vi "PH_Beckhoff_StepMot.constructor.vi"(0 "name":string, 2 "data in":string, 5 "error in(no error)":errorcluster) -> (14 "i ref out":refnum<vi>, 16 "data out":string, 19 "error out":errorcluster)   [LabVIEW 2014, in "PH_Beckhoff_StepMot.lvlib"]
doc: "This is the constructor of a class.\n\nLicense Agreement for this software:\n\nCopyright (C)\nGesellschaft für Schwerionenforschung, GSI\nPlanckstr. 1\n64291 Darmstadt\nGermany\n\nContact: D.Beck@gsi.de \n\nThis program is free software; you can redistribute it and/or modify it under the terms of the \nGNU General Public License as published by the Free Software Foundation; either version 2 of \nthe license, or (at your option) any later version.\n\nThis program is distributed in the hope that it will be useful, but WITHOUT ANY WARRANTY; \nwithout even the implied warranty of MERCHANTABILITY or FITNESS FOR A PARTICULAR PURPOSE. See the GNU General License for more details (http://www.gnu.org).\n\nGesellschaft für Schwerionenforschung, GSI\nPlanckstr. 1, 64291 Darmstadt, Germany\nFor all questions and ideas contact: M.Richter@gsi.de, H.Brand@gsi.de or D.Beck@gsi.de.\nLast update: 16-JUN-2004"
uses:
  PH_Beckhoff_StepMot.lvlib
  PH_Beckhoff_StepMot.i attribute.ctl
  PH_Beckhoff_StepMot.Axis Cluster.ctl
  instr.lib/Beckhoff/Specials/Step Motor Klemmen/Beckhoff.Step Motor - Motor Configuration.ctl
  instr.lib/Beckhoff/Read and Write Register/Step Motor Klemmen/Beckhoff.Step Motor - Feature Register 1.ctl
  instr.lib/Beckhoff/Read and Write Register/Step Motor Klemmen/Beckhoff.Step Motor - Feature Register 2.ctl
  PH_Beckhoff/PH_Beckhoff.lvlib
  PH_Basics/PH_Stepmotor_BaseClass/PH_Stepmotor_BaseClass.lvlib
  instr.lib/Beckhoff/Beckhoff - Driver np.lvlib
  CS_Core/CSSystem/CSSystemLib/CSSystemLib.lvlib
  PH_Basics/PH_Class/PH_Class.lvlib
  PH_Basics/PH_Common/PH_Common.lvlib
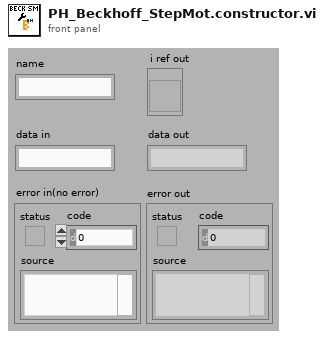
[diagram p1: front panel]
types:
  T1 = typedef "PH_Beckhoff_StepMot.lvlib/PH_Beckhoff_StepMot.i attribute.ctl" = cluster{"Axes Settings":T2[], "GUI Refs":cluster{"Axes Settings":refnum<vi>, "Stati":refnum<vi>}, "Get Beckhoff Settings":bool}
  T2 = typedef "PH_Beckhoff_StepMot.lvlib/PH_Beckhoff_StepMot.Axis Cluster.ctl" = cluster{"Step Motor Configuration":T3, "To set?":bool, "Endswitch inverted?":bool}
  T3 = typedef "Beckhoff - Driver np.lvlib/Beckhoff.Step Motor - Motor Configuration.ctl" = cluster{"Feature Register":T4, "I max A [mA]":dbl, "I max B [mA]":dbl, "v min":u32, "v max":u32, "a max":u32, "I hold [%]":u32, "Steps/qp":u32, "Feature Register 2":T5}
  T4 = typedef "Beckhoff - Driver np.lvlib/Beckhoff.Step Motor - Feature Register 1.ctl" = cluster{"en Auto Start":bool, "en Auto Stop":bool, "dis Wd Timer":bool, "OP Mode 1":bool, "OP Mode 2":bool, "Ramp Type":bool, "inv Pos Feedback":bool, "en User Cur Table":bool, "en Latch Evt Clr Pos":bool, "en Multi Latch Vals":bool, "en Sign Disp*":bool, "Feedback Type*":bool, "en neg Gate Lock*":bool, "en pos Gate Lock*":bool, "dis Enc Fltr*":bool, "en Counter Mode*":bool}
  T5 = typedef "Beckhoff - Driver np.lvlib/Beckhoff.Step Motor - Feature Register 2.ctl" = cluster{"rev Homing Dir":bool, "en Decac Ramp":bool, "Latch Reg Pos":bool, "Show Idle":bool, "dis Ref Input 1":bool, "dis Ref Input 2":bool, "en ext Auto Start":bool, "N/A":bool, "N/A":bool, "N/A":bool, "N/A":bool, "N/A":bool, "en Clr Proc Data":bool, "en Man Ecl Tolerce*":bool, "rev Dig Input 1":bool, "rev Dig Input 2":bool}
  T6 = enum16{"SetAttribute", "GetAttribute", "CreateAttribute", "DestroyAttribute", "DestroyAllAtributes"}
  T7 = typedef "PH_Beckhoff.lvlib/PH_Beckhoff.constructor Data in.ctl" = cluster{"Default Values":T8, "Description":string, "Hardware configured?":bool, "Activate Change Manager?":bool, "Difference to handle an analog input as change":u32}
  T8 = typedef "PH_Beckhoff.lvlib/PH_Beckhoff.Values.ctl" = cluster{"Sonderklemmen Inputs":T9, "Analog Inputs":T10, "Analog Outputs":T12, "Digital Inputs":T13, "Digital Outputs":T14}
  T9 = typedef "PH_Beckhoff.lvlib/PH_Beckhoff.Sonderklemmen Inputs.ctl" = cluster{"Total Length":u32, "Name":string, "Value":u64, "Quality":bool, "Service ID":i32, "Offset":u32, "Length":u32}[]
  T10 = typedef "PH_Beckhoff.lvlib/PH_Beckhoff.Analog Inputs.ctl" = cluster{"Name":string, "Value":u32, "Quality":bool, "Service ID":i32, "Sca Type":T11}[]
  T11 = typedef "PH_Beckhoff.lvlib/PH_Beckhoff.Scaling Type.ctl" = enum16{"none", "0 ... 15 Bit -> 0 ... 5", "0 ... 15 Bit -> 0 ... 10", "0 ... 15 Bit -> 0 ... 25", "0 ... 15 Bit -> 4 ... 20", "0 ... 15 Bit -> 0 ... 1", "0 ... 15 Bit -> 0 ... 20000", "0 ... 15 Bit -> 0 ... 24000"}
  T12 = typedef "PH_Beckhoff.lvlib/PH_Beckhoff.Analog Outputs.ctl" = cluster{"Name":string, "Value":u32, "Quality":bool, "Wanted Value":u32, "Service ID":i32, "Sca Type":T11}[]
  T13 = typedef "PH_Beckhoff.lvlib/PH_Beckhoff.Digital Inputs.ctl" = cluster{"Name":string, "Value":bool, "Quality":bool, "Service ID":i32, "inverted?":bool}[]
  T14 = typedef "PH_Beckhoff.lvlib/PH_Beckhoff.Digital Outputs.ctl" = cluster{"Name":string, "Value":bool, "Quality":bool, "Wanted Value":bool, "Service ID":i32, "inverted?":bool}[]
  T15 = typedef "PH_Stepmotor_BaseClass.lvlib/PH_Stepmotor_BaseClass.i attribute.ctl" = cluster{"Device Error":errorcluster, "Axes PSDB Thread":cluster{"Ref":refnum<vi>, "Q-Ref":refnum<queue>, "Data Status":T16}, "Axes":T17[], "Axes PSDB Infos":cluster{"GUI Name":string, "PSDB Instance ID":i32, "PSDB Status Service ID":i32, "Axis":i32, "Class":string}[], "GUI Refs":T22}
  T16 = typedef "PH_PSDBWriter.lvlib/PH_PSDBWriter.Data Status.ctl" = i16
  T17 = typedef "PH_Stepmotor_BaseClass.lvlib/PH_Stepmotor_BaseClass.Axis Attributes.ctl" = cluster{"Settings":T18, "Endswitch?":bool, "DIM Service IDs":T20, "Activity":T21, "Configured?":bool, "Position":cluster{"Current":i32, "Target":i32}, "Position to set":cluster{"New?":bool, "Wanted":i32}, "Stop?":bool, "Reset?":bool, "Move?":bool, "Nothing connected?":bool}
  T18 = typedef "PH_Stepmotor_BaseClass.lvlib/PH_Stepmotor_BaseClass.Axis Settings.ctl" = cluster{"Sign change":bool, "Width":dbl, "Calibration":dbl, "Unit":string, "Motor Type":T19, "Unit Width":string, "Unit CF":string}
  T19 = typedef "PH_Stepmotor_BaseClass.lvlib/PH_Stepmotor_BaseClass.Motor Type.ctl" = enum16{"Unspecific", "OWIS 49.120.2633", "OWIS 49.060.1033", "OWIS 43.040.2558", "Diamond Motion 2200 series", "OWIS 49.120.266B.MV6", "Calorimeter", "Linear Stage 1", "MICOS VT-80", "MICOS VT-80 S", "Standa Rotstage nt0.95A", "PUF RA 320.200", "PUF RA 800.200", "PUF RA 800.400", "PUF RA 400.50", "1324.nn.800.50", "1324.n9c.800.50", "1324.nn.320.200", "1324.nn.400.200", "1324.nn.800.200", "1324.nn.400.50", "1324.8c9c.800.50", "1324.8c9c.400.200"}
  T20 = typedef "PH_Stepmotor_BaseClass.lvlib/PH_Stepmotor_BaseClass.Axis DIM Service IDs.ctl" = cluster{"Settings":i32, "Information":i32}
  T21 = typedef "PH_Stepmotor_BaseClass.lvlib/PH_Stepmotor_BaseClass.Axis Activity.ctl" = enum16{"No Information", "stopped", "running", "Failure", "Alarm", "stopped at backward ES", "stopped at foreward ES"}
  T22 = typedef "PH_Stepmotor_BaseClass.lvlib/PH_Stepmotor_BaseClass.GUI Refs.ctl" = cluster{"Axes Configuration":refnum<vi>, "Device Error":refnum<vi>, "Axes PSDB Infos":refnum<vi>}
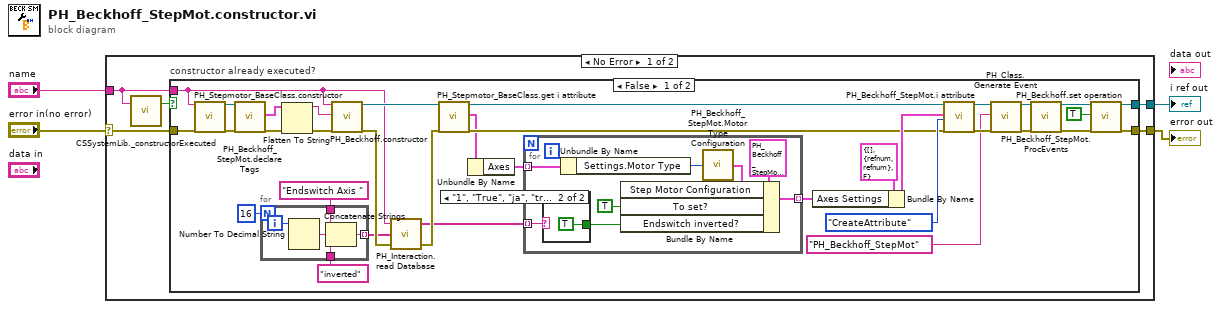
[diagram p0: block diagram]
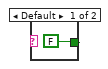
[diagram p2: hidden frame]
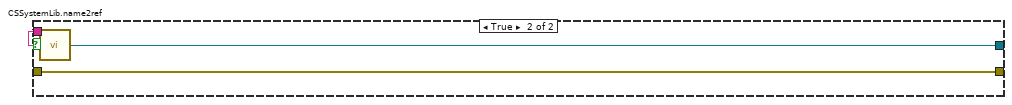
[diagram p3: hidden frame]
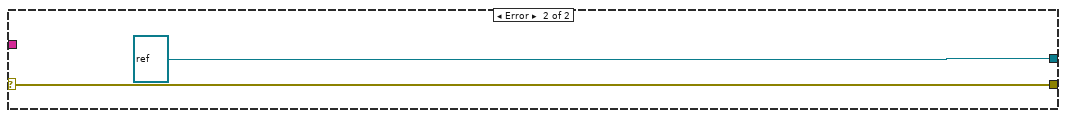
[diagram p4: hidden frame]
diagram:
  n1 = case shown="No Error" "error in(no error)" {
    selector: "error in(no error)" -> [w7 w63]
    tunnel: "name" -> [w6 _]
    tunnel: [w9 refnum<vi> refnum ("obj refnum")] -> w3
    tunnel: [w8 w63] -> w2
    frame No Error {
      n2 = call "CSSystemLib._constructorExecuted.vi"("name"=w6) -> ("constructor executed?"=w5:bool)  [unwired: 18 in]
      n3 = case "constructor already executed?" shown="False" w5 {
        tunnel: [w34 w59] -> w9
        tunnel: [w33 w61] -> w8
        tunnel: w7 -> [w21 w61]
        tunnel: w6 -> [w14 w60]
        frame False {
          n4 = call "PH_Stepmotor_BaseClass.constructor.vi"("name"=w14, "error in"=w21) -> ("i ref out"=w23:refnum<vi>, "error out"=w22:errorcluster)  [unwired: 15 in, 1 out]
          n5 = call "PH_Beckhoff_StepMot.declare Tags.vi"("i ref in"=w23, "error in (no error)"=w22) -> ("Data in cluster"=w40:T7, "error out"=w39:errorcluster)  [unwired: 15 in, 1 out]
          n6 = for {
            N: 16 -> [_]
            tunnel: [w46] -> w12 mode=indexing
            tunnel: "Endswitch Axis " -> [w45]
            tunnel: "inverted" -> [w44]
            i -> [w48]
            n7 = Number To Decimal String(number=w48) -> (decimal integer string=w47:string)  [unwired: 1 in]
            n8 = Concatenate Strings(w45, w47, w44) -> (w46:string)
          }
          n9 = Flatten To String(anything=w40, error in (no error)=w39) -> (data string=w42:string, error out=w43:errorcluster)  [unwired: 2 in, 1 out]
          n10 = call "PH_Beckhoff.constructor.vi"("name"=w14, "data in"=w42, "error in(no error)"=w43) -> ("i ref out"=w19:refnum<vi>, "error out"=w30:errorcluster)  [unwired: 14 in, 1 out]
          n11 = call "PH_Interaction.read Database.vi"("error in (no error)"=w30, "Strings to search for"=w12, "DB Entry to read"=w14) -> ("error out"=w16:errorcluster, "Values"=w15:string[])  [unwired: 1 in]
          n12 = call "PH_Stepmotor_BaseClass.get i attribute.vi"("i ref in"=w19, "error in (no error)"=w16) -> ("i ref out"=w18:refnum<vi>, "i attribute"=w17:T15, "error out"=w20:errorcluster)  [unwired: 15 in]
          n13 = Unbundle By Name(w17) -> ("Axes"=w38:T17[])
          n14 = for {
            tunnel: w38 -> [w56] mode=indexing
            tunnel: [w54] -> w35 mode=indexing
            tunnel: w15 -> [w50] mode=indexing
            n15 = case shown="\"1\", \"True\", \"ja\", \"true\"" w50 {
              tunnel: [FALSE TRUE] -> w49
              frame Default {
              }
              frame "1", "True", "ja", "true" {
              }
            }
            n16 = Unbundle By Name(w56) -> ("Settings.Motor Type"=w53:T19)
            n17 = call "PH_Beckhoff_StepMot.Motor Type Configuration.vi"("Motor Type"=w53) -> ("Step Motor Configuration"=w52:T3)
            n18 = Bundle By Name(cluster=T2 {"Step Motor Configuration"={"Feature Register"={"en Auto Start"=FALSE, "en Auto Stop"=FALSE, "dis Wd Timer"=FALSE, "OP Mode 1"=FALSE, "OP Mode 2"=FALSE, "Ramp Type"=FALSE, "inv Pos Feedback"=FALSE, "en User Cur Table"=FALSE, "en Latch Evt Clr Pos"=FALSE, "en Multi Latch Vals"=FALSE, "en Sign Disp*"=FALSE, "Feedback Type*"=FALSE, "en neg Gate Lock*"=FALSE, "en pos Gate Lock*"=FALSE, "dis Enc Fltr*"=FALSE, "en Counter Mode*"=FALSE}, "I max A [mA]"=0.0, "I max B [mA]"=0.0, "v min"=0, "v max"=0, "a max"=0, "I hold [%]"=0, "Steps/qp"=0, "Feature Register 2"={"rev Homing Dir"=FALSE, "en Decac Ramp"=FALSE, "Latch Reg Pos"=FALSE, "Show Idle"=FALSE, "dis Ref Input 1"=FALSE, "dis Ref Input 2"=FALSE, "en ext Auto Start"=FALSE, "N/A"=FALSE, "N/A"=FALSE, "N/A"=FALSE, "N/A"=FALSE, "N/A"=FALSE, "en Clr Proc Data"=FALSE, "en Man Ecl Tolerce*"=FALSE, "rev Dig Input 1"=FALSE, "rev Dig Input 2"=FALSE}}, "To set?"=FALSE, "Endswitch inverted?"=FALSE} ("Klemmenset"), "Step Motor Configuration"=w52, "To set?"=TRUE, "Endswitch inverted?"=w49) -> (w54:T2)
          }
          n19 = Bundle By Name(cluster=T1 {"Axes Settings"=[], "GUI Refs"={"Axes Settings"=refnum, "Stati"=refnum}, "Get Beckhoff Settings"=FALSE} ("CLASS.i attribute"), "Axes Settings"=w35) -> (w36:T1)
          n20 = call "PH_Beckhoff_StepMot.i attribute.vi"("VI Refnum"=w18, "CLASS.i attribute"=w36, "Action"=T6."CreateAttribute", "error in (no error)"=w20) -> ("VI Refnum out"=w24:refnum<vi>, "error out"=w32:errorcluster)  [unwired: 13 in, 1 out]
          n21 = call "PH_Class.Generate Event.vi"("i ref in"=w24, "Class"="PH_Beckhoff_StepMot", "error in (no error)"=w32) -> ("i ref out"=w25:refnum<vi>, "error out"=w26:errorcluster)  [unwired: 15 in]
          n22 = call "PH_Beckhoff_StepMot.ProcEvents.vi"("i ref in"=w25, "error in"=w26) -> ("i ref out"=w28:refnum<vi>, "error out"=w27:errorcluster)  [unwired: 16 in]
          n23 = call "PH_Beckhoff.set operation.vi"("VI in"=w28, "operation?"=TRUE, "error in (no error)"=w27) -> ("VI out"=w34:refnum<vi>, "error out"=w33:errorcluster)  [unwired: 15 in]
        }
        frame True {
          n24 = call "CSSystemLib.name2ref.vi"("name"=w60) -> ("obj refnum"=w59:refnum<vi>)
        }
      }
    }
    frame Error {
    }
  }
  "i ref out" <- w3
  "error out" <- w2
